vi "resizable_alert_Recolor Splitters.vi"(10 "hide":bool, 11 "VI reference":refnum<vi>) -> ()   [LabVIEW 2020]
doc: "Change the colors of any splitter bars on a VI's panel to hide or show them. When showing them, use color to visualize run-time sizing behavior."
uses:
  <vilib>/Utility/miscctls.llb/LVForegroundBackgroundColorsTypeDef.ctl
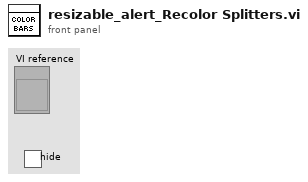
[diagram p1: front panel]
types:
  T1 = typedef "LVForegroundBackgroundColorsTypeDef.ctl" = cluster{"Foreground Color":u32, "Background Color":u32}
  T2 = enum16{"Sticks Top/Left", "Sticks Bottom/Right", "Proportional"}
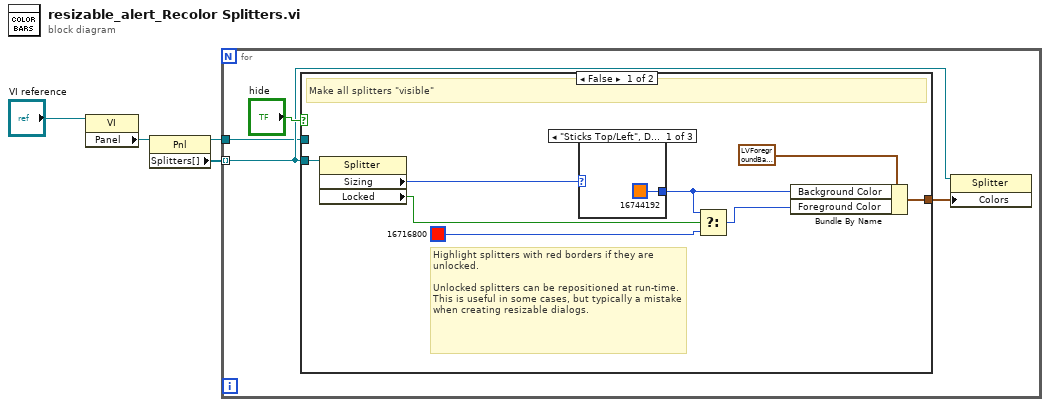
[diagram p0: block diagram]
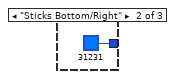
[diagram p2: hidden frame]
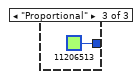
[diagram p3: hidden frame]
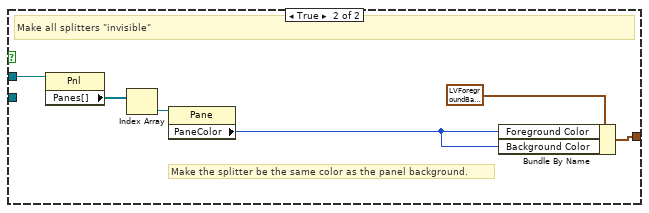
[diagram p4: hidden frame]
diagram:
  n1 = property class="VI"(reference="VI reference") -> ("Panel"=w3:refnum<vi>)  [unwired: 1 in, 2 out]
  n2 = property class="Pnl"(reference=w3) -> (reference out=w1:refnum<vi>, "Splitters[]"=w4:refnum<vi>[])  [unwired: 1 in, 1 out]
  n3 = for {
    tunnel: w4 -> [w6] mode=indexing
    tunnel: w1 -> [w5]
    n4 = case shown="False" "hide" {
      tunnel: [w15 w24] -> w7
      tunnel: w6 -> [w14 _]
      tunnel: w5 -> [_ w22]
      frame False {
        # "Highlight splitters with red borders if they are unlocked.\n\nUnlocked splitters can be repositioned at run-time. This is useful in some cases, but typically a mistake when creating resizable dialogs."
        # "Make all splitters \"visible\""
        n5 = property class="Splitter"(reference=w14) -> ("Sizing"=w13:T2, "Locked"=w12:bool)  [unwired: 1 in, 2 out]
        n6 = case shown="\"Sticks Top/Left\", Default" w13 {
          tunnel: [u32 16744192 ("Foreground Color") u32 31231 ("Foreground Color") u32 11206513 ("Foreground Color")] -> w9
          frame "Sticks Top/Left", Default {
          }
          frame "Sticks Bottom/Right" {
          }
          frame "Proportional" {
          }
        }
        n7 = Select(t=w9, s=w12, f=u32 16716800 ("Foreground Color")) -> (s? t:f=w11:u32)
        n8 = Bundle By Name(cluster=T1 {"Foreground Color"=12369084, "Background Color"=12369084} ("Colors"), "Background Color"=w9, "Foreground Color"=w11) -> (w15:T1)
      }
      frame True {
        # "Make the splitter be the same color as the panel background."
        # "Make all splitters \"invisible\""
        n9 = property class="Pnl"(reference=w22) -> ("Panes[]"=w21:refnum<vi>[])  [unwired: 1 in, 2 out]
        n10 = Index Array(array=w21) -> (element=w23:refnum<vi>)  [unwired: 1 in]
        n11 = property class="Pane"(reference=w23) -> ("PaneColor"=w20:u32)  [unwired: 1 in, 2 out]
        n12 = Bundle By Name(cluster=T1 {"Foreground Color"=16777238, "Background Color"=16777238} ("Colors"), "Foreground Color"=w20, "Background Color"=w20) -> (w24:T1)
      }
    }
    n13 = property class="Splitter"(reference=w6, "Colors"=w7) -> ()  [unwired: 1 in, 2 out]
  }
